vi "Graph_Controls_Ctrl_Index.vi"(5 "OldVal":variant, 11 "NewVal":variant) -> (4 "Control Ref OUT":refnum<vi>, 8 "Graph Tools Out":T1={"Zoom Out"=FALSE, "Zoom In"=FALSE, "Reset Zoom"=FALSE, "Pan Tool"=FALSE, "Show Cursor"=FALSE, "Load File"=FALSE, "Fit Tool"=FALSE, "Smooth Tool"=FALSE, "Merge Tool"=FALSE, "Auto Scale"=FALSE, "Apply Color"=FALSE, "Color Map"=enum."Fire"})   [LabVIEW 2014]
uses:
  Type Defs/STED Graph Controls.ctl
panel:
  in  "STED Graph Tools Data Type":T1={"Zoom Out"=FALSE, "Zoom In"=FALSE, "Reset Zoom"=FALSE, "Pan Tool"=FALSE, "Show Cursor"=FALSE, "Load File"=FALSE, "Fit Tool"=FALSE, "Smooth Tool"=FALSE, "Merge Tool"=FALSE, "Auto Scale"=FALSE, "Apply Color"=FALSE, "Color Map"=enum."Fire"}
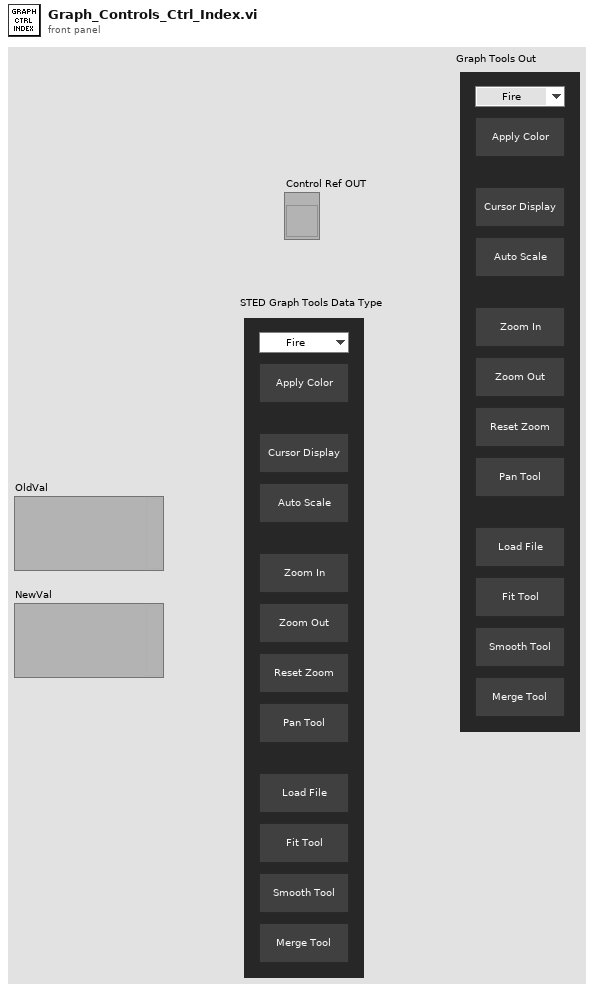
[diagram p1: front panel]
types:
  T1 = typedef "STED Graph Controls.ctl" = cluster{"Zoom Out":bool, "Zoom In":bool, "Reset Zoom":bool, "Pan Tool":bool, "Show Cursor":bool, "Load File":bool, "Fit Tool":bool, "Smooth Tool":bool, "Merge Tool":bool, "Auto Scale":bool, "Apply Color":bool, "Color Map":enum16{"System", "Fire", "Gray", "Red", "Green", "Blue", "Cyan", "Magenta", "Yellow", "Red-White", "Green-White", "Blue-White", "Glow"}}
  T2 = cluster{"Zoom Out":bool, "Zoom In":bool, "Reset Zoom":bool, "Pan Tool":bool, "Show Cursor":bool, "Load File":bool, "Fit Tool":bool, "Smooth Tool":bool, "Merge Tool":bool, "Auto Scale":bool, "Apply Color":bool, "Color Map":bool}
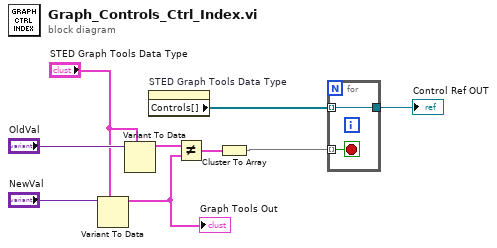
[diagram p0: block diagram]
diagram:
  n1 = Variant To Data(type="STED Graph Tools Data Type", Variant="NewVal") -> (data=w2:T1)  [unwired: 1 in, 1 out]
  "Graph Tools Out" <- w2
  n2 = Variant To Data(type="STED Graph Tools Data Type", Variant="OldVal") -> (data=w5:T1)  [unwired: 1 in, 1 out]
  n3 = property on="STED Graph Tools Data Type" class="Clust (strict)"() -> ("Controls[]"=w1:refnum<vi>[])  [unwired: 2 in, 2 out]
  n4 = Not Equal?(x=w5, y=w2) -> (x != y?=w9:T2)
  n5 = Cluster To Array(cluster=w9) -> (array=w6:bool[])
  n6 = for {
    tunnel: w6 -> [w10] mode=indexing
    tunnel: w1 -> [w11] mode=indexing
    tunnel: [w11] -> w4
    stop <- w10 stop-if-true
  }
  "Control Ref OUT" <- w4
